vi "top_stack.vi"(9 "pilha input":T1[](array[typedef])) -> (1 "top":T1)   [LabVIEW 2017]
uses:
  segment.ctl
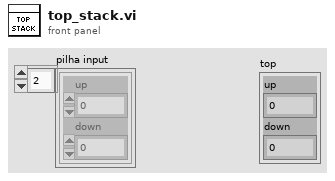
[diagram p1: front panel]
types:
  T1 = typedef "segment.ctl" = cluster{"up":dbl, "down":dbl}
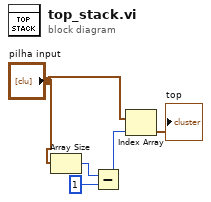
[diagram p0: block diagram]
diagram:
  n1 = Array Size(array="pilha input") -> (size(s)=w5:i32)
  n2 = Subtract(x=w5, y=1) -> (x-y=w2:i32)
  n3 = Index Array(array="pilha input", index=w2) -> (element=→"top":T1)
